vi "cs-scanning_altztrig.vi"() -> ()   [LabVIEW 2017]
uses:
  controls/boolean_info.ctl
  z-axis-params.ctl
  <vilib>/rvi/Emulation/niFpgaGetClockAttributes.vi
  <vilib>/rvi/Emulation/niFpgaSctlEmulationGetInTimedLoop.vi
  <vilib>/rvi/Emulation/niFpgaEmulationReportErrorSimple.vi
  <vilib>/rvi/Emulation/niFpgaProcessEmulError.vi
  <vilib>/rvi/eio/common/nirviEmuTemplateMethod_errors.vi
  <vilib>/rvi/Emulation/niFpgaEmulationIsFPGAContextNoSignature.vi
  <vilib>/rvi/DataTransferAndStorage/Container/Common/niFpgaContainerGetUniqueNameForEmu.vi
  <vilib>/rvi/Memory/Memory_Emulation/niFpgaMemoryEmulationCacheClearOnFirstRun.vi
  <vilib>/rvi/Memory/Memory_Emulation/nirvimemoryEmulationManagerCache_MakeExclusive.vi
  <vilib>/rvi/Memory/Memory_Emulation/niFpgaMemoryEmulationValidateCache.vi
  <vilib>/rvi/Memory/Memory_Emulation/nirvimemoryEmulationManagerCache_InsertValue.vi
  <vilib>/Utility/error.llb/Clear Errors.vi
  <vilib>/rvi/Memory/Memory_Emulation/nirvimemoryEmulationManagerCache_ReleaseExclusive.vi
  <vilib>/rvi/Memory/Memory_Emulation/nirvimemoryEmulationManagerCache_GetValue.vi
  <vilib>/rvi/Memory/Memory_Emulation/nirvimemoryEmulationManagerCache_SetValue.vi
  <vilib>/rvi/Emulation/niFpgaCriticalErrorInLSC.vi
  <vilib>/eio/EIONode/EIONode.xnode
  <vilib>/rvi/DataTransferAndStorage/Container/XNode/niFpgaContainer.xnode
  <vilib>/rvi/DataTransferAndStorage/Register/Emulation/niFpgaRegisterEmulation.vi
  FPGA-data-logging.lvlib
  libimaging-cs.lvlib
panel:
  in  "Kiz_down":sgl format="%#_13g"
  in  "max_Z_settle_samples":i16
  in  "do_Alt_Ztrigger":bool
  in  "step_down_frac":fxp<+,8,1>
  out "state1-count":u64
  out "state5-count":u64
  out "state4-count":u64
  out "state3-count":u64
  out "state2-count":u64
  in  "collect all":bool
  in  "collect move":bool=TRUE
  out "iter":i32
  out "entity-index":i16
  in  "TsTicks":u32=1600
  in  "z-axis-params":T1={"TOL"=0.3, "ramp_rate"=0.0, "z_u_max"=5.0, "setpoint"=0.0, "Ki"=0.001, "Z_error_threshold"=0.0, "Z_settled_samples_threshold "=0, "z_UP"=0.0, "zup_N"=0, "TF Order"=2, "Num"=[-0.00254, 0.000408, 0.00295, 0.0, 0.0, 0.0, 0.0, 0.0, 0.0], "Den"=[0.982758, -1.98194, 1.0, 0.0, 0.0, 0.0, 0.0, 0.0, 0.0]} {"Z_error_threshold" format="%#_13g"; "ramp_rate" format="%#_13g"; "TOL" format="%#_13g"}
  out "number-settled-samples-Z":i16
  out "Current Case":i16
  out "boolean \nindicators":T2
  out "z-u(k)":sgl
  in  "ABORT":bool
  out "read fifo timeout":bool
  in  "numEntities":i16
  in  "init Z up":fxp<+/-,16,5>
  in  "trigger-0":bool
  out "number-settled-samples-y":i16
  out "number-settled-samples-x":i16
  in  "xy-error-threshold":sgl format="%#_13g"
  in  "settled-samples\nthreshold":i16
  in  "Ki-xy":sgl=0.001 format="%#_13g"
  in  "xy-bound":sgl
  in  "initial case":i16
  # "- If collect all = fasle and collect move = false,\nwe only collect measurement data.\n- If collect all = false, and collect move = true,\nwe collect measurement and move data.\n- If collect all = true, we collect everything."
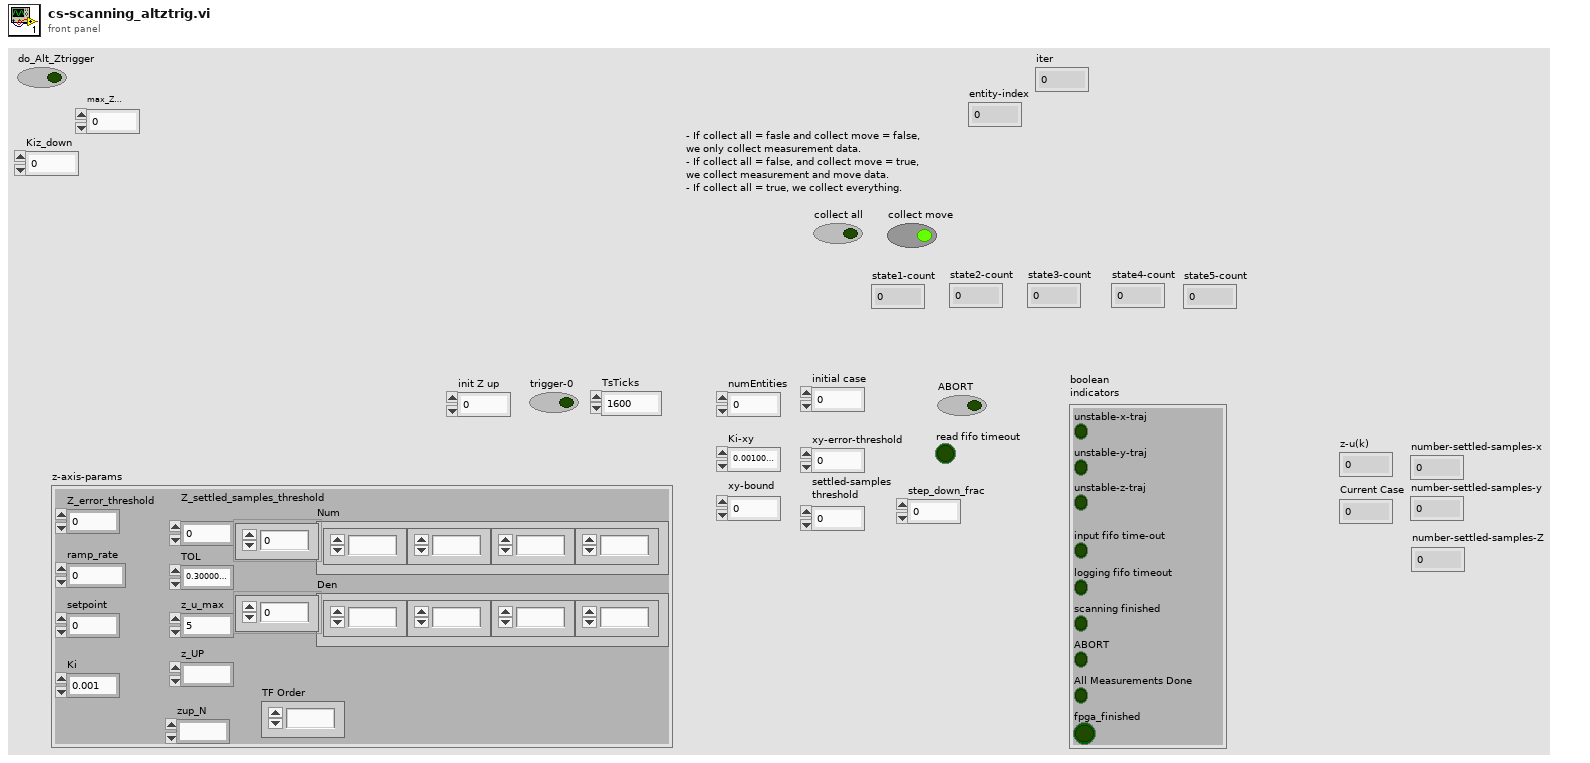
[diagram p1: front panel]
types:
  T1 = typedef "z-axis-params.ctl" = cluster{"TOL":sgl, "ramp_rate":sgl, "z_u_max":sgl, "setpoint":sgl, "Ki":sgl, "Z_error_threshold":sgl, "Z_settled_samples_threshold ":i16, "z_UP":fxp<+/-,16,5>, "zup_N":i16, "TF Order":i32, "Num":sgl[], "Den":sgl[]}
  T2 = typedef "boolean_info.ctl" = cluster{"unstable-z-traj":bool, "input fifo time-out":bool, "logging fifo timeout":bool, "scanning finished":bool, "unstable-x-traj":bool, "unstable-y-traj":bool, "ABORT":bool, "All Measurements Done":bool, "fpga_finished":bool}
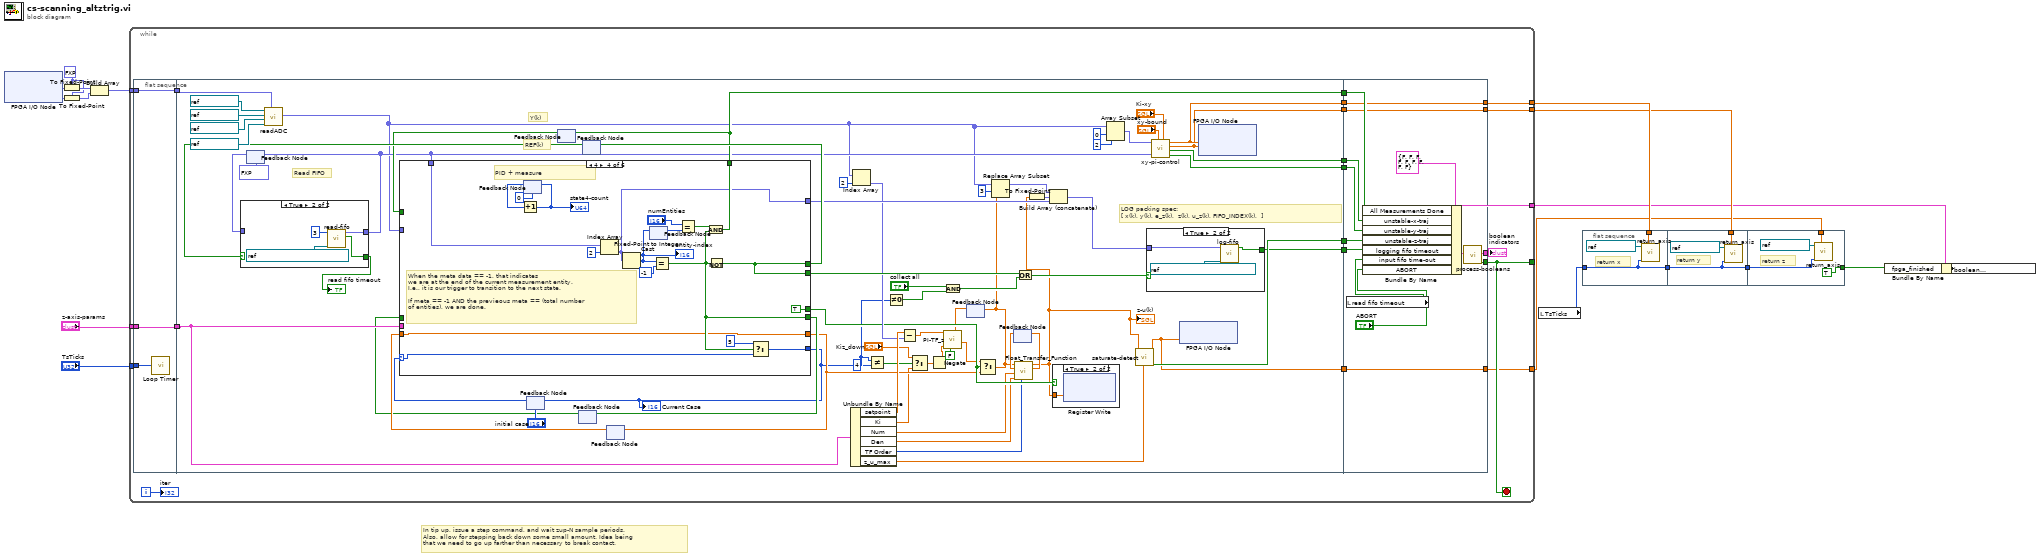
[diagram p0: block diagram]
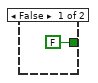
[diagram p3: hidden frame]
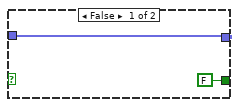
[diagram p4: hidden frame]
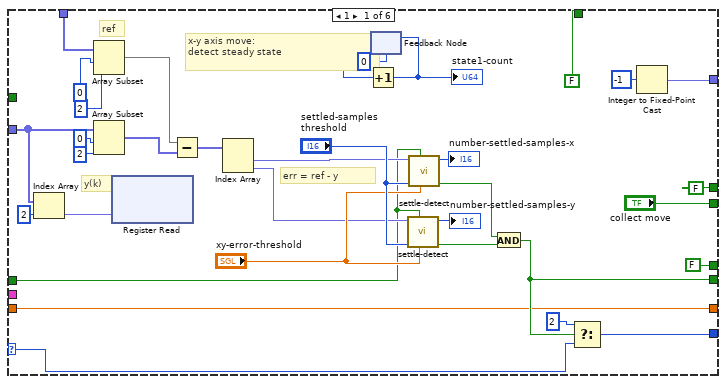
[diagram p5: hidden frame]
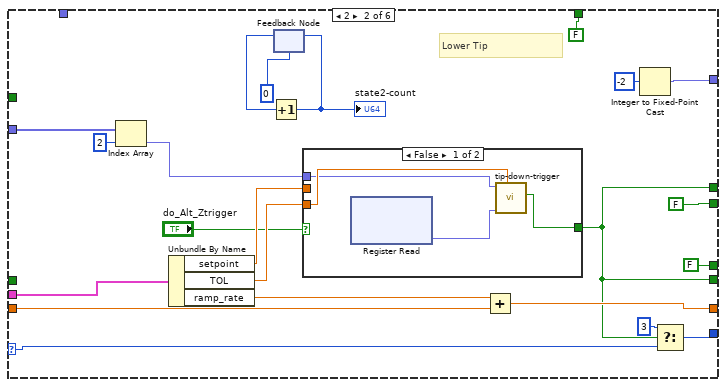
[diagram p6: hidden frame]
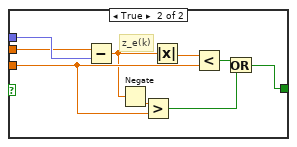
[diagram p7: hidden frame]
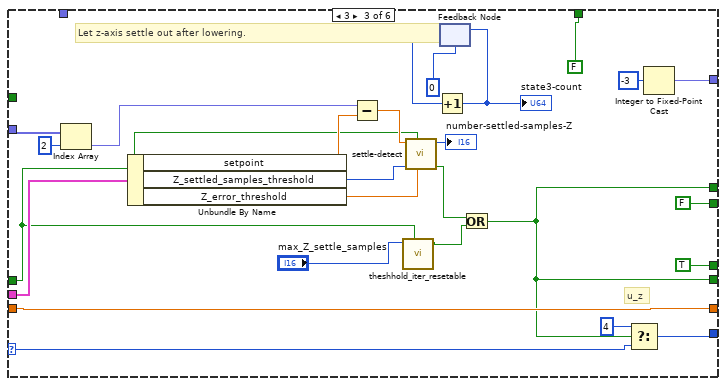
[diagram p8: hidden frame]
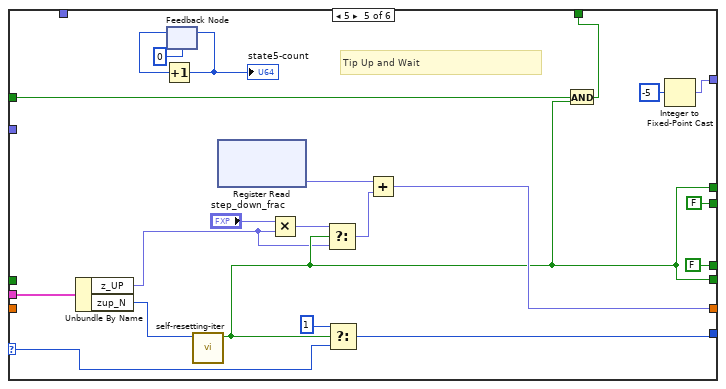
[diagram p9: hidden frame]
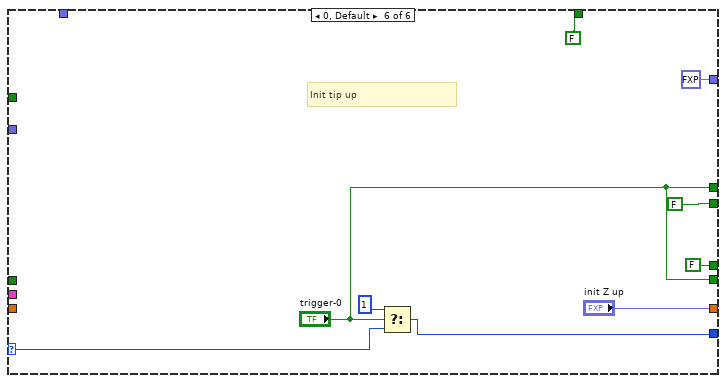
[diagram p10: hidden frame]
diagram:
  w12 = fxp<+/-,16,5> 0.0 ("fixed-point type")
  # "In tip up, issue a step command, and wait zup-N sample periods.\nAlso, allow for stepping back down some small amount. Idea being \nthat we need to go up farther than necessary to break contact."
  n1 = xnode "FPGA I/O Node"() -> ("Mod2/AI0"=w15:fxp<+/-,24,5>, "Mod2/AI1"=w13:fxp<+/-,24,5>)  [unwired: 2 in, 2 out]
  n2 = To Fixed-Point(fixed-point type=w12, number=w15) -> (fixed-point=w17:fxp<+/-,16,5>)
  n3 = To Fixed-Point(fixed-point type=w12, number=w13) -> (fixed-point=w14:fxp<+/-,16,5>)
  n4 = Build Array(w17, w14) -> (w16:fxp<+/-,16,5>[])
  n5 = while {
    tunnel: w16 -> [w29]
    tunnel: "z-axis-params" -> [w28]
    tunnel: "TsTicks" -> [w27]
    tunnel: [w26] -> _
    tunnel: [w24] -> w6
    tunnel: [w22] -> w5
    tunnel: [w20] -> w4
    tunnel: [w18] -> w3
    i -> [w19]
    stop <- w26 stop-if-true
    n6 = flat-sequence {
      tunnel: w29 -> [w39]
      tunnel: [w39] -> w36
      tunnel: w27 -> [w37]
      tunnel: w28 -> [w38]
      tunnel: [w38] -> w35
      tunnel: w36 -> [w103]
      tunnel: w35 -> [w84]
      tunnel: [w95] -> w34
      tunnel: [w94] -> w33
      tunnel: [w93] -> w32
      tunnel: [w92] -> w31
      tunnel: [w73] -> w30
      tunnel: [w87] -> w25
      tunnel: [w86] -> w23
      tunnel: [w85] -> w21
      tunnel: w34 -> [w274]
      tunnel: w33 -> [w273]
      tunnel: w32 -> [w272]
      tunnel: w31 -> [w269]
      tunnel: w30 -> [w266]
      tunnel: [w265] -> w26
      tunnel: [w264] -> w18
      tunnel: w25 -> [w263]
      tunnel: [w263] -> w24
      tunnel: w23 -> [w262]
      tunnel: [w262] -> w22
      tunnel: [w261] -> w20
      tunnel: w21 -> [w261]
      frame #0 {
        n7 = call "Loop Timer"("Count(Ticks)"=w37) -> ()  [unwired: 1 out]
      }
      frame #1 {
        # "REF(k)"
        # "Y(k)"
        # "LOG packing spec:\n[ x(k), y(k), e_z(k),  z(k), u_z(k), FIFO_INDEX(k),  ]"
        # "Read FIFO"
        n8 = feedback #1(fxp<+/-,16,5>[] [0.0, 0.0, 0.0] ("unpacked-data")) -> (w98:fxp<+/-,16,5>[])
        n9 = call "readADC.vi"("x(0), y(0)"=w103, "z-height"=refnum<k21> "Mod2/AI3" ("y - ADC"), "z-err- ADC"=refnum<k21> "Mod2/AI2" ("y - ADC"), "y - ADC"=refnum<k21> "Mod2/AI1", "x - ADC"=refnum<k21> "Mod2/AI0") -> ("x_y_ze_z_k"=w55:fxp<+/-,17,6>[])  [unwired: 6 in]
        n10 = feedback #2("initial case") -> (w104:i16)
        n11 = feedback #3() -> (w83:bool)  [unwired: 1 in]
        n12 = feedback #4() -> (w81:bool)  [unwired: 1 in]
        n13 = feedback #5() -> (w89:bool)  [unwired: 1 in]
        n14 = case shown="True" w89 {
          tunnel: w98 -> [w112 _]
          tunnel: [w112 w114] -> w70
          tunnel: [FALSE ("timout?") w113] -> w91
          frame False {
          }
          frame True {
            n15 = call "read-fifo.vi"("FIFO In"=refnum<k21> "host-to-fpga-fxp-16-5", "numChan"=3) -> ("timout?"=w113:bool, "unpacked-data"=w114:fxp<+/-,16,5>[])  [unwired: 8 in]
          }
        }
        "read fifo timeout" <- w91
        n16 = feedback-in #1(w70) -> ()
        n17 = feedback #6() -> (w97:sgl)  [unwired: 1 in]
        n18 = case shown="4" w104 {
          selector: w104 -> [w142 w171 w204 w228 w250 w258]
          tunnel: ["collect move" FALSE FALSE ("trigger-0") w220 FALSE FALSE] -> w76
          tunnel: [w143 w166 w205 w229 w249 w260] -> w51
          tunnel: w55 -> [w117 w168 w209 _ _ _]
          tunnel: [FALSE w153 w189 w220 w235 "trigger-0"] -> w90
          tunnel: [w122 w157 w191 w212 w239 "init Z up"] -> w56
          tunnel: w97 -> [w122 w164 w191 w212 _ _]
          tunnel: w84 -> [_ w170 w202 _ w246 _]
          tunnel: [FALSE FALSE FALSE w219 w231 FALSE] -> w73
          tunnel: w70 -> [w133 _ _ w222 _ _]
          tunnel: w83 -> [_ _ _ _ w244 _]
          tunnel: w81 -> [w131 _ w186 _ _ _]
          tunnel: [w129 w153 w189 w218 w235 "trigger-0"] -> w82
          tunnel: [FALSE ("trigger-0") FALSE ("trigger-0") TRUE ("trigger-0") TRUE ("trigger-0") FALSE ("trigger-0") FALSE ("trigger-0")] -> w68
          tunnel: [w120 w154 w193 w213 w233 fxp<+/-,16,5> 0.0 ("Element")] -> w74
          frame 1 {
            # "y(k)"
            # "err = ref - y"
            # "ref"
            # "x-y axis move: \ndetect steady state"
            n19 = Index Array(array=w117, index=2) -> (element=w119:fxp<+/-,17,6>)
            n20 = Array Subset(array=w133, index=0, length=2) -> (w137:fxp<+/-,16,5>[])
            n21 = Array Subset(array=w117, index=0, length=2) -> (w136:fxp<+/-,17,6>[])
            n22 = xnode ("Register Read")("Data"=w119) -> ()  [unwired: 1 in, 1 out]
            n23 = Subtract(x=w137, y=w136) -> (x-y=w128:fxp<+/-,18,7>[])
            n24 = Index Array(array=w128) -> (element #1=w135:fxp<+/-,18,7>, element #2=w134:fxp<+/-,18,7>)  [unwired: 2 in]
            n25 = feedback #7(u64 0) -> (w125:u64)
            n26 = Increment(x=w125) -> (x+1=w126:u64)
            "state1-count" <- w126
            n27 = feedback-in #7(w126) -> ()
            n28 = call "settle-detect.vi"("error-max"="xy-error-threshold", "reset"=w131, "settled-samples\nthreshold"="settled-samples\nthreshold", "err(k)"=w134) -> ("has-settled"=w150:bool, "number-settled-samples"=→"number-settled-samples-y":u16)  [unwired: 6 in]
            n29 = call "settle-detect.vi"("error-max"="xy-error-threshold", "reset"=w131, "settled-samples\nthreshold"="settled-samples\nthreshold", "err(k)"=w135) -> ("has-settled"=w149:bool, "number-settled-samples"=→"number-settled-samples-x":u16)  [unwired: 6 in]
            n30 = And(x=w149, y=w150) -> (x .and. y?=w129:bool)
            n31 = Select(t=i16 2, s=w129, f=w142) -> (s? t:f=w143:i16)
            n32 = Integer to Fixed-Point Cast(integer=i16 -1) -> (fixed-point=w120:fxp<+/-,16,5>)  [unwired: 1 in]
          }
          frame 2 {
            # "Lower Tip"
            n33 = Index Array(array=w168, index=2) -> (element=w167:fxp<+/-,17,6>)
            n34 = Unbundle By Name(w170) -> ("setpoint"=w156:sgl, "TOL"=w152:sgl, "ramp_rate"=w172:sgl)
            n35 = feedback #8(u64 0) -> (w160:u64)
            n36 = Increment(x=w160) -> (x+1=w161:u64)
            "state2-count" <- w161
            n37 = feedback-in #8(w161) -> ()
            n38 = case shown="False" "do_Alt_Ztrigger" {
              tunnel: w167 -> [w173 w185]
              tunnel: w156 -> [_ w184]
              tunnel: [w175 w181] -> w153
              tunnel: w152 -> [w174 w179]
              frame False {
                n39 = xnode ("Register Read")() -> ("Data"=w176:fxp<+/-,16,5>)  [unwired: 1 in, 1 out]
                n40 = call "tip-down-trigger.vi"("TOL"=w174, "Vo"=w176, "e(k)"=w173) -> ("trigger"=w175:bool)  [unwired: 8 in]
              }
              frame True {
                # "z_e(k)"
                n41 = Subtract(x=w184, y=w185) -> (x-y=w177:sgl)
                n42 = Negate(x=w177) -> (-x=w178:sgl)
                n43 = Greater?(x=w178, y=w179) -> (0:w180:bool)
                n44 = Absolute Value(x=w177) -> (abs(x)=w183:sgl)
                n45 = Less?(x=w183, y=w179) -> (x < y?=w182:bool)
                n46 = Or(x=w182, y=w180) -> (x .or. y?=w181:bool)
              }
            }
            n47 = Add(x=w172, y=w164) -> (x+y=w157:sgl)
            n48 = Integer to Fixed-Point Cast(integer=i16 -2) -> (fixed-point=w154:fxp<+/-,16,5>)  [unwired: 1 in]
            n49 = Select(t=i16 3, s=w153, f=w171) -> (s? t:f=w166:i16)
          }
          frame 3 {
            # "u_z"
            # "Let z-axis settle out after lowering."
            n50 = Index Array(array=w209, index=2) -> (element=w207:fxp<+/-,17,6>)
            n51 = Unbundle By Name(w202) -> ("setpoint"=w192:sgl, "Z_settled_samples_threshold"=w201:i16, "Z_error_threshold"=w200:sgl)
            n52 = Subtract(x=w207, y=w192) -> (x-y=w210:sgl)
            n53 = call "theshhold_iter_resetable.vi"("reset"=w186, "N"="max_Z_settle_samples") -> ("Boolean"=w188:bool)  [unwired: 8 in, 1 out]
            n54 = call "settle-detect.vi"("error-max"=w200, "reset"=w186, "settled-samples\nthreshold"=w201, "err(k)"=w210) -> ("has-settled"=w190:bool, "number-settled-samples"=→"number-settled-samples-Z":u16)  [unwired: 6 in]
            n55 = feedback #9(u64 0) -> (w197:u64)
            n56 = Increment(x=w197) -> (x+1=w198:u64)
            "state3-count" <- w198
            n57 = feedback-in #9(w198) -> ()
            n58 = Or(x=w190, y=w188) -> (x .or. y?=w189:bool)
            n59 = Select(t=i16 4, s=w189, f=w204) -> (s? t:f=w205:i16)
            n60 = Integer to Fixed-Point Cast(integer=i16 -3) -> (fixed-point=w193:fxp<+/-,16,5>)  [unwired: 1 in]
          }
          frame 4 {
            # "When the meta data == -1, that indicates\nwe are at the end of the current measurement entity.\nI.e., it is our trigger to transition to the next state.\n\nIf meta == -1 AND the previeous meta == (total number\nof entities), we are done."
            # "PID + measure"
            n61 = feedback #10(u64 0) -> (w216:u64)
            n62 = Increment(x=w216) -> (x+1=w217:u64)
            "state4-count" <- w217
            n63 = feedback-in #10(w217) -> ()
            n64 = Index Array(array=w222, index=2) -> (element=w213:fxp<+/-,16,5>)
            n65 = Fixed-Point to Integer Cast(1:w213) -> (0:w221:i16)
            "entity-index" <- w221
            n66 = feedback #11() -> (w223:i16)  [unwired: 1 in]
            n67 = feedback-in #11(w221) -> ()
            n68 = Equal?(x=w221, y=i16 -1) -> (x = y?=w218:bool)
            n69 = Equal?(x="numEntities", y=w223) -> (x = y?=w224:bool)
            n70 = And(x=w224, y=w218) -> (x .and. y?=w219:bool)
            n71 = Not(x=w218) -> (.not. x?=w220:bool)
            n72 = Select(t=i16 5, s=w218, f=w228) -> (s? t:f=w229:i16)
          }
          frame 5 {
            # "Tip Up and Wait"
            n73 = Unbundle By Name(w246) -> ("z_UP"=w234:fxp<+/-,16,5>, "zup_N"=w245:i16)
            n74 = feedback #12(u64 0) -> (w242:u64)
            n75 = Increment(x=w242) -> (x+1=w243:u64)
            "state5-count" <- w243
            n76 = feedback-in #12(w243) -> ()
            n77 = call "self-resetting-iter.vi"("N"=w245) -> ("Boolean"=w235:bool)  [unwired: 9 in, 1 out]
            n78 = xnode ("Register Read")() -> ("Data"=w247:fxp<+/-,16,5>)  [unwired: 1 in, 1 out]
            n79 = Multiply(x="step_down_frac", y=w234) -> (x*y=w238:fxp<+/-,24,6>)
            n80 = Select(t=w238, s=w235, f=w234) -> (s? t:f=w236:fxp<+/-,24,6>)
            n81 = Select(t=i16 1, s=w235, f=w250) -> (s? t:f=w249:i16)
            n82 = Add(x=w247, y=w236) -> (x+y=w239:fxp<+/-,25,7>)
            n83 = And(x=w244, y=w235) -> (x .and. y?=w231:bool)
            n84 = Integer to Fixed-Point Cast(integer=i16 -5) -> (fixed-point=w233:fxp<+/-,16,5>)  [unwired: 1 in]
          }
          frame 0, Default {
            # "Init tip up"
            n85 = Select(t=i16 1, s="trigger-0", f=w258) -> (s? t:f=w260:i16)
          }
        }
        "Current Case" <- w51
        n86 = feedback-in #2(w51) -> ()
        n87 = feedback-in #3(w73) -> ()
        n88 = feedback-in #4(w82) -> ()
        n89 = feedback-in #5(w90) -> ()
        n90 = feedback-in #6(w56) -> ()
        n91 = Unbundle By Name(w84) -> ("setpoint"=w72:sgl, "Ki"=w45:sgl, "Num"=w67:sgl[], "Den"=w66:sgl[], "TF Order"=w64:i32, "z_u_max"=w65:sgl)
        n92 = Index Array(array=w55, index=2) -> (element=w69:fxp<+/-,17,6>)
        n93 = Not Equal?(x=w51, y=i16 4) -> (x != y?=w48:bool)
        n94 = Not Equal To 0?(x=w51) -> (x != 0?=w79:bool)
        n95 = Subtract(x=w72, y=w69) -> (x-y=w61:sgl)
        n96 = Select(t="Kiz_down", s=w48, f=w45) -> (s? t:f=w47:sgl)
        n97 = Negate(x=w47) -> (-x=w46:sgl)
        n98 = And(x="collect all", y=w79) -> (x .and. y?=w77:bool)
        n99 = feedback #13() -> (w57:sgl)  [unwired: 1 in]
        n100 = call "PI-TF_z.vi"("u(k-1)"=w57, "reset"=FALSE, "Ki"=w46, "e(k)"=w61) -> ("u(k)"=w59:sgl)  [unwired: 7 in]
        n101 = Select(t=w59, s=w68, f=w56) -> (s? t:f=w52:sgl)
        n102 = feedback-in #13(w52) -> ()
        n103 = Replace Array Subset(array=w55, new element=w52, index=3) -> (w54:fxp<+/-,17,6>[])
        n104 = feedback #14() -> (w62:sgl[])  [unwired: 1 in]
        n105 = call "Float_Transfer_Function.vi"("TF Order"=w64, "Den"=w66, "Num"=w67, "State In"=w62, "Input"=w52) -> ("State Out"=w63:sgl[], "Output"=w58:sgl)  [unwired: 4 in]
        "z-u(k)" <- w58
        n106 = feedback-in #14(w63) -> ()
        n107 = Or(x=w76, y=w77) -> (x .or. y?=w80:bool)
        n108 = To Fixed-Point(number=w58) -> (fixed-point=w75:fxp<+/-,16,5>)  [unwired: 1 in]
        n109 = Build Array (concatenate)(w54, w75, w74) -> (w96:fxp<+/-,17,6>[])
        n110 = case shown="True" w68 {
          tunnel: w58 -> [_ w106]
          frame False {
          }
          frame True {
            n111 = xnode ("Register Write")("Data"=w106) -> ()  [unwired: 1 in, 1 out]
          }
        }
        n112 = Array Subset(array=w55, index=0, length=2) -> (w40:fxp<+/-,17,6>[])
        n113 = call "saturate-detect.vi"("bound"=w65, "x"=w58) -> ("saturated"=w93:bool, "sat(x)"=w85:sgl)  [unwired: 8 in]
        n114 = case shown="True" w80 {
          tunnel: w96 -> [_ w109]
          tunnel: [FALSE ("logging-timeout?") w108] -> w92
          frame False {
          }
          frame True {
            n115 = call "log-fifo.vi"("FIFO In"=refnum<k21> "fpga-to-host2-fxp-16-5", "input-data"=w109) -> ("logging-timeout?"=w108:bool)  [unwired: 9 in]
          }
        }
        n116 = call "xy-pi-control.vi"("Ki-xy"="Ki-xy", "xy-umax"="xy-bound", "xy-ref"=w70, "x_k-y_k"=w40) -> ("u_y saturated"=w94:bool, "u_x saturated"=w95:bool, "sat(u_y)"=w86:sgl, "sat(u_x)"=w87:sgl)  [unwired: 4 in]
        n117 = xnode "FPGA I/O Node"("Mod1/AO2"=w85) -> ()  [unwired: 1 in, 1 out]
        n118 = xnode "FPGA I/O Node"("Mod1/AO0"=w87, "Mod1/AO1"=w86) -> ()  [unwired: 2 in, 2 out]
      }
      frame #2 {
        n119 = local read "read fifo timeout"() -> (w268:bool)
        n120 = Bundle By Name(cluster=T2 {"unstable-z-traj"=FALSE, "input fifo time-out"=FALSE, "logging fifo timeout"=FALSE, "scanning finished"=FALSE, "unstable-x-traj"=FALSE, "unstable-y-traj"=FALSE, "ABORT"=FALSE, "All Measurements Done"=FALSE, "fpga_finished"=FALSE} ("boolean errors"), "All Measurements Done"=w266, "unstable-x-traj"=w274, "unstable-y-traj"=w273, "unstable-z-traj"=w272, "logging fifo timeout"=w269, "input fifo time-out"=w268, "ABORT"="ABORT") -> (w270:T2)
        n121 = call "process-booleans.vi"("boolean indicators 2"=w270) -> ("scaning finished"=w265:bool, "boolean indicators"=w264:T2)  [unwired: 9 in]
      }
    }
    "boolean \nindicators" <- w18
    "iter" <- w19
  }
  n122 = local read "TsTicks"() -> (w7:u32)
  n123 = flat-sequence {
    tunnel: w7 -> [w276]
    tunnel: w6 -> [w277]
    tunnel: [w276] -> w9
    tunnel: w5 -> [w280]
    tunnel: w9 -> [w278]
    tunnel: [w278] -> w8
    tunnel: w4 -> [w284]
    tunnel: w8 -> [w282]
    tunnel: [TRUE] -> w2
    frame #0 {
      # "return x"
      n124 = call "return_axis.vi"("u(0)"=w277, "TsTicks"=w276, "FPGA I/O In"=refnum<k21> "Mod1/AO0") -> ()  [unwired: 9 in]
    }
    frame #1 {
      # "return y"
      n125 = call "return_axis.vi"("u(0)"=w280, "TsTicks"=w278, "FPGA I/O In"=refnum<k21> "Mod1/AO1") -> ()  [unwired: 9 in]
    }
    frame #2 {
      # "return z"
      n126 = call "return_axis.vi"("u(0)"=w284, "TsTicks"=w282, "FPGA I/O In"=refnum<k21> "Mod1/AO2") -> ()  [unwired: 9 in]
    }
  }
  n127 = Bundle By Name(cluster=w3, "fpga_finished"=w2) -> (w1:T2)
  n128 = local write "boolean \nindicators"(w1) -> ()
